vi "ProgressBar-Call logging progress window.vi"(8 "error in (no error)":errorcluster, 11 "Z-stack queue cluster":T1={"Imaging Protocol"=enum."Live Imaging", "Number of Trials"=0, "Frame Size"=512, "# Averaged frames"=0, "Dwell time (us)"=0.0, "Index of Z-plane"=0, "Timelapse?"=FALSE, "Logging process is active"=FALSE, "Speed logging enabled"=FALSE, "tdms file ref"=refnum, "path"=path "", "Trial Number"=0, "Expected # points acquired"=FALSE, "Manually stopped"=FALSE, "Last trial"=FALSE, "Ch0 data"=[], "Ch1 data"=[], "Ref Data"=[], "Ref Frame Time"=[], "Image Time"=[], "Continuous Time"=[], "Ref X Length"=0, "Ref Y Length"=0, "# Ref Averaged frames"=0, "Ref Dwell time (us)"=0.0, "Points acquired"={"Ch0 last trial"=0, "Ch1 last trial"=0, "All trials"=0}, "HW Timings File"=refnum} {"Ref Dwell time (us)" format="%#.6g"; "Frame Size" items=["100X100"=100, "128X128"=128, "200X200"=200, "256X256"=256, "512X512"=512, "1024x1024"=1024, "2048x2048"=2048]; "Dwell time (us)" format="%#.6g"}) -> (0 "error out":errorcluster)   [LabVIEW 2020]
uses:
  Typedefs/Logging queue element.ctl
  Typedefs/Imaging Protocols enum.ctl
  Typedefs/Frame Size.ctl
  Typedefs/Acquired points count.ctl
  Global Variables/General Globals.vi
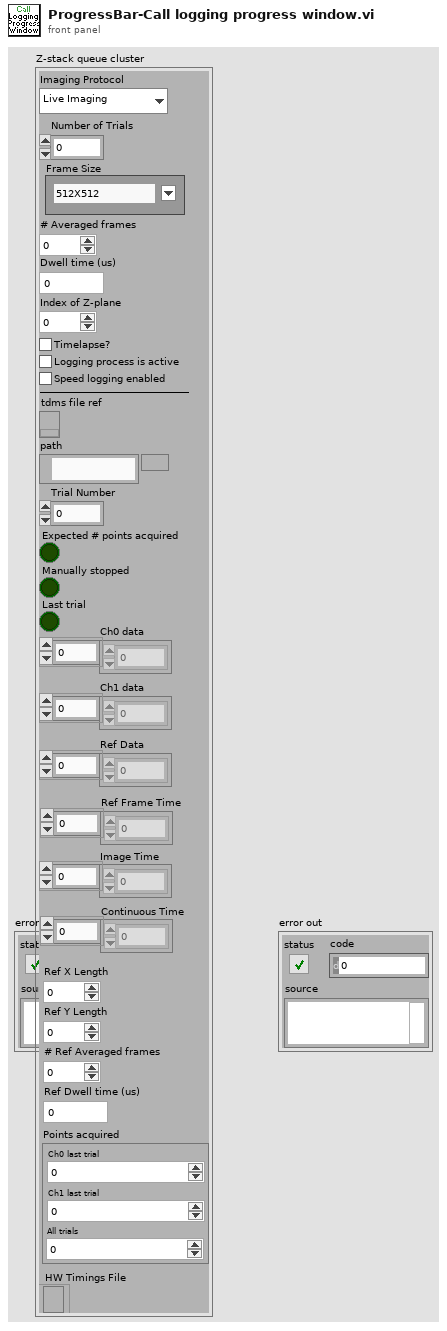
[diagram p1: front panel]
types:
  T1 = typedef "Logging queue element.ctl" = cluster{"Imaging Protocol":T2, "Number of Trials":u16, "Frame Size":T3, "# Averaged frames":u16, "Dwell time (us)":dbl, "Index of Z-plane":i32, "Timelapse?":bool, "Logging process is active":bool, "Speed logging enabled":bool, "tdms file ref":refnum<k34>, "path":path, "Trial Number":i32, "Expected # points acquired":bool, "Manually stopped":bool, "Last trial":bool, "Ch0 data":u32[], "Ch1 data":u32[], "Ref Data":u32[], "Ref Frame Time":u64[], "Image Time":u64[], "Continuous Time":u64[], "Ref X Length":u16, "Ref Y Length":u16, "# Ref Averaged frames":u16, "Ref Dwell time (us)":dbl, "Points acquired":T4, "HW Timings File":refnum<file>}
  T2 = typedef "Imaging Protocols enum.ctl" = enum16{"AOL Z-Stack", "Motor Z Stack", "Functional Acquisition", "Single Plane Acquisition", "Volume Acquisition", "Live Imaging", "Live Plane Imaging", "Live Volume Imaging"}
  T3 = typedef "Frame Size.ctl" = u16
  T4 = typedef "Acquired points count.ctl" = cluster{"Ch0 last trial":u64, "Ch1 last trial":u64, "All trials":u64}
  T5 = typedef "Progress bar window values input cluster.ctl" = cluster{"Total":i32, "Current":i32, "Message in":string, "Sender":enum16{"Acquisition", "Logging", "File gen"}}
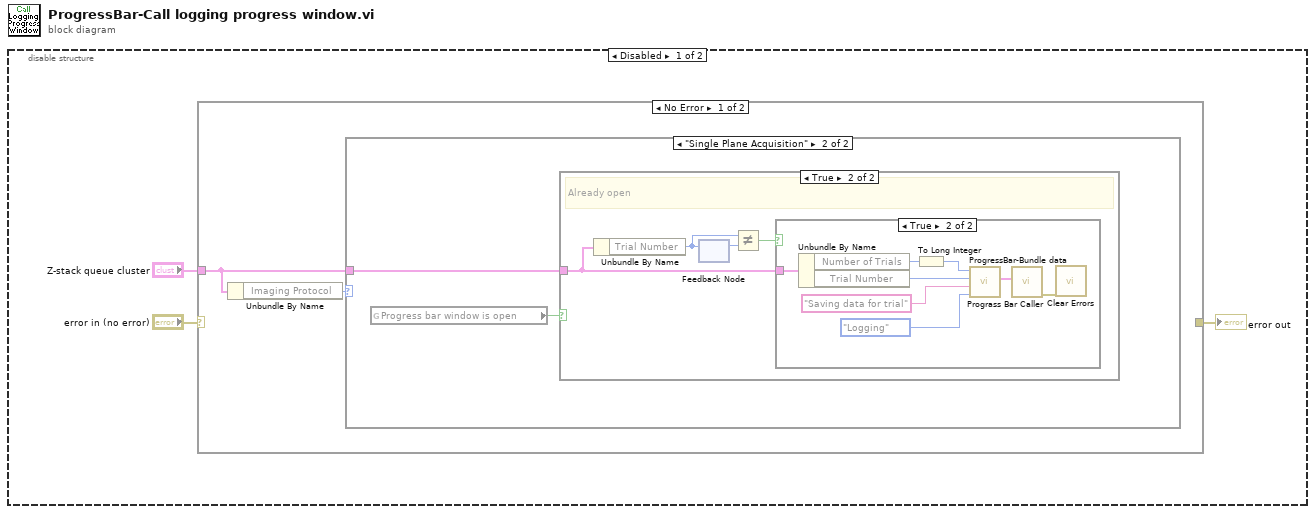
[diagram p0: block diagram]
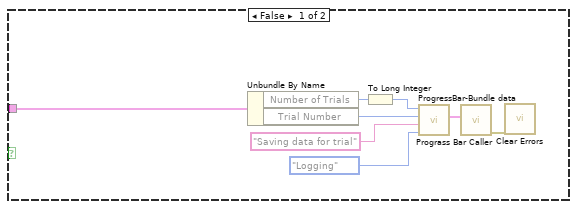
[diagram p3: hidden frame]
diagram:
  n1 = disable-structure shown="Disabled" {
    frame Disabled {
      n2 = case shown="No Error" "error in (no error)" {
        selector: "error in (no error)" -> [_ w28]
        tunnel: "Z-stack queue cluster" -> [w5 _]
        tunnel: [_ w28] -> w1
        frame No Error {
          n3 = Unbundle By Name(w5) -> ("Imaging Protocol"=w4:T2)
          n4 = case shown="\"Single Plane Acquisition\"" w4 {
            tunnel: w5 -> [_ w7]
            frame Default {
            }
            frame "Single Plane Acquisition" {
              n5 = global read "General Globals.vi" "Progress bar window is open"() -> (w6:bool)
              n6 = case shown="True" w6 {
                tunnel: w7 -> [w14 w19]
                frame False {
                  n7 = Unbundle By Name(w14) -> ("Number of Trials"=w15:u16, "Trial Number"=w13:i32)
                  n8 = To Long Integer(number=w15) -> (32bit integer=w9:i32)
                  n9 = call "ProgressBar-Bundle data.vi"("Sender"=enum16{"Acquisition", "Logging", "File gen"}."Logging", "Message in"="Saving data for trial" ("string"), "Current"=w13, "Total"=w9) -> ("Progress bar window values input"=w12:T5)  [unwired: 7 in]
                  n10 = call "Prograss Bar Caller.vi"("Progress bar window values input"=w12) -> ("error out"=w10:errorcluster)  [unwired: 10 in]
                  n11 = call <vilib>:"Clear Errors.vi"("error in (no error)"=w10) -> ()  [unwired: 6 in, 1 out]
                }
                frame True {
                  # "Already open"
                  n12 = Unbundle By Name(w19) -> ("Trial Number"=w17:i32)
                  n13 = feedback-in #1(w17) -> ()
                  n14 = feedback #1() -> (w18:i32)  [unwired: 1 in]
                  n15 = Not Equal?(x=w17, y=w18) -> (x != y?=w16:bool)
                  n16 = case shown="True" w16 {
                    tunnel: w19 -> [_ w26]
                    frame False {
                    }
                    frame True {
                      n17 = Unbundle By Name(w26) -> ("Number of Trials"=w27:u16, "Trial Number"=w20:i32)
                      n18 = To Long Integer(number=w27) -> (32bit integer=w22:i32)
                      n19 = call "ProgressBar-Bundle data.vi"("Sender"=enum16{"Acquisition", "Logging", "File gen"}."Logging", "Message in"="Saving data for trial" ("string"), "Current"=w20, "Total"=w22) -> ("Progress bar window values input"=w25:T5)  [unwired: 7 in]
                      n20 = call "Prograss Bar Caller.vi"("Progress bar window values input"=w25) -> ("error out"=w23:errorcluster)  [unwired: 10 in]
                      n21 = call <vilib>:"Clear Errors.vi"("error in (no error)"=w23) -> ()  [unwired: 6 in, 1 out]
                    }
                  }
                }
              }
            }
          }
        }
        frame Error {
        }
      }
      "error out" <- w1
    }
    frame Enabled {
    }
  }
